vi "CreateErrorReporter.vi"(8 "error in":errorcluster, 9 "default reporting parameter":T1, 10 "reporting parameters":T1[](array[typedef]), 11 "message ref in":refnum<class "CLM_PriorityLocalMessage.lvclass">) -> (0 "error out":errorcluster, 3 "error reporter out":refnum<class "ErrorReporter.lvclass">)   [LabVIEW 2013, in "CLM_ErrorHandler.lvlib" / "ErrorReporter.lvclass"]
uses:
  ErrorReporter.lvclass
  ReportingParameter.ctl
  <vilib>/CLM/LocalMessenger/PriorityLocalMessage/CLM_PriorityLocalMessage.lvclass
  ErrorReporter.lvclass/ErrorReporter.ctl
  Var_SetMultReportingParameters.vi
  Var_SetReportingParameter.vi
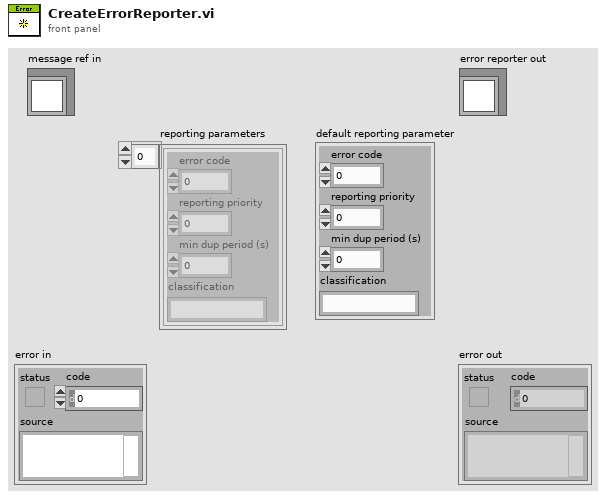
[diagram p1: front panel]
types:
  T1 = typedef "CLM_ErrorHandler.lvlib/ErrorReporter.lvclass/ReportingParameter.ctl" = cluster{"error code":i32, "reporting priority":i32, "min dup period (s)":dbl, "classification":string}
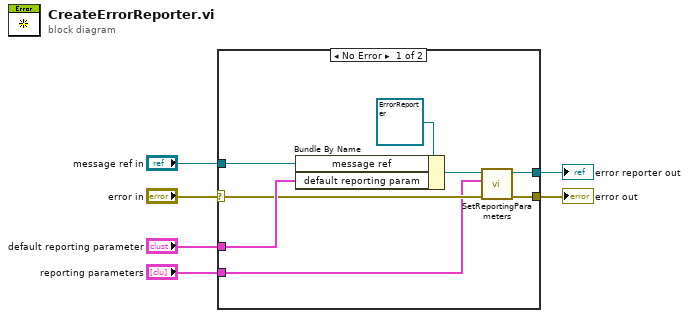
[diagram p0: block diagram]
diagram:
  n1 = case shown="No Error" "error in" {
    selector: "error in" -> [w12 w15]
    tunnel: [w10 w15] -> w5
    tunnel: "message ref in" -> [w11 _]
    tunnel: [w8 _] -> w4
    tunnel: "default reporting parameter" -> [w13 _]
    tunnel: "reporting parameters" -> [w7 _]
    frame No Error {
      n2 = Bundle By Name(cluster=refnum<class "ErrorReporter.lvclass"> refnum ("ErrorReporter out"), "message ref"=w11, "default reporting param"=w13) -> (w9:refnum<class "ErrorReporter.lvclass">)
      n3 = call "SetReportingParameters.vi"("error in"=w12, "reporting parameters"=w7, "error reporter in"=w9) -> ("error out"=w10:errorcluster, "error reporter out"=w8:refnum<class "ErrorReporter.lvclass">)  [unwired: 7 in]
    }
    frame Error {
    }
  }
  "error out" <- w5
  "error reporter out" <- w4
